vi "ZenReport init.vi"(8 "error IO":errorcluster, 9 "Get part / batch data":variant, 11 "Report type":string(combo)="Part") -> (0 "Error out":errorcluster, 3 "output cluster":T1)   [LabVIEW 2015]
uses:
  Typedefs/ZenReport internal data.ctl
  Typedefs/System configuration.ctl
  Typedefs/Part configuration.ctl
  Typedefs/Batch configuration.ctl
  Typedefs/Internal data.ctl
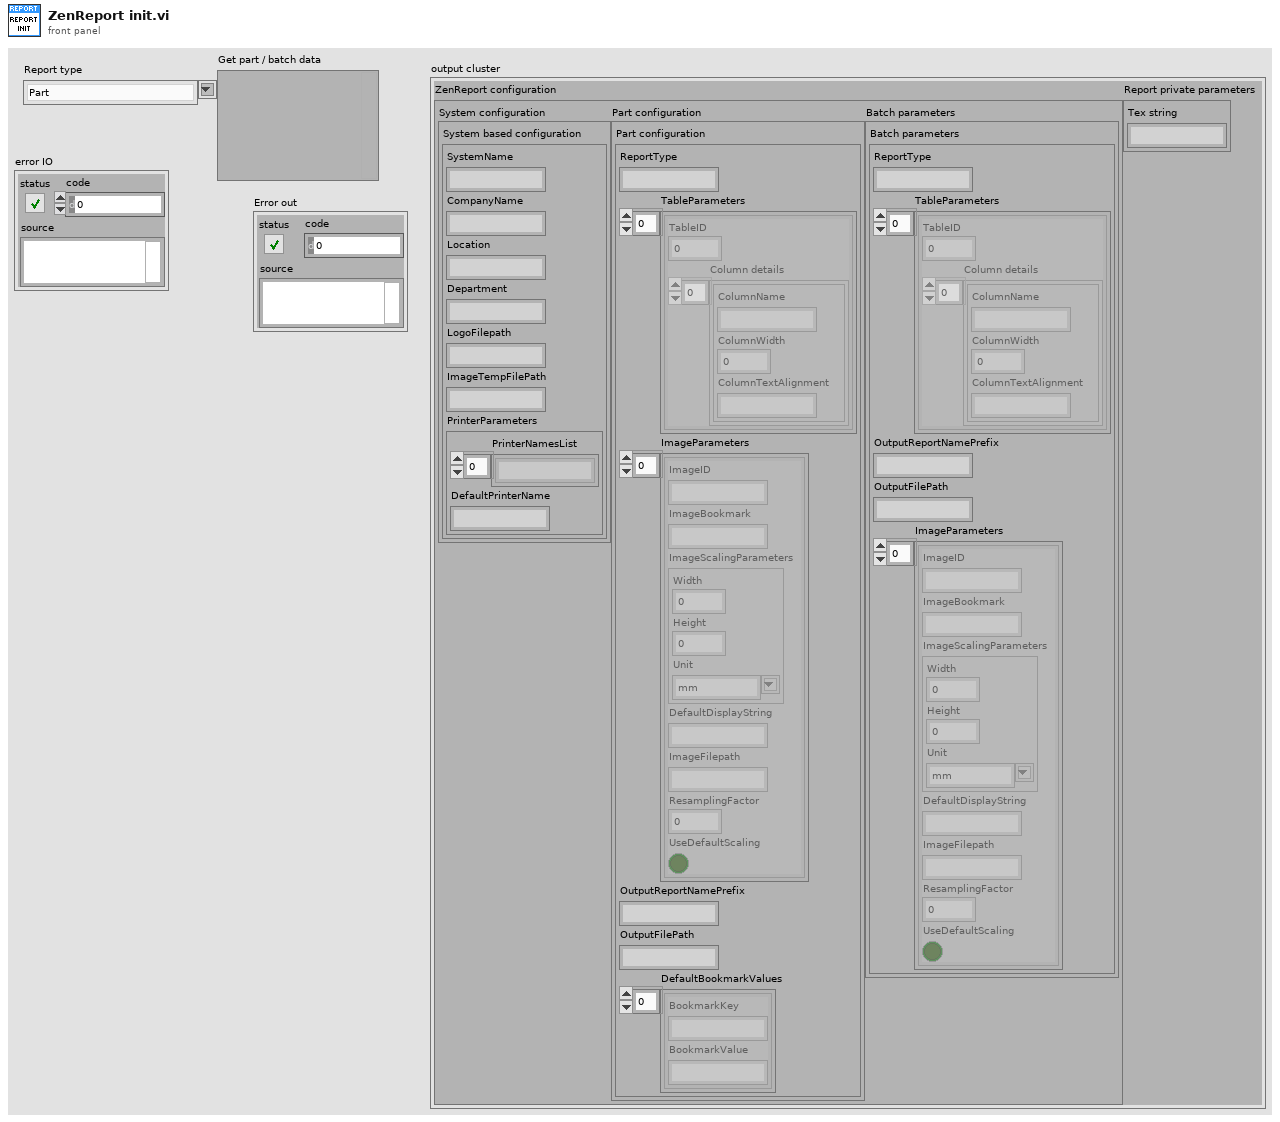
[diagram p1: front panel]
types:
  T1 = typedef "ZenReport internal data.ctl" = cluster{"ZenReport configuration":cluster{"System configuration":T2, "Part configuration":T3, "Batch parameters":T4}, "Report private parameters":T5}
  T2 = typedef "System configuration.ctl" = cluster{"System based configuration":cluster{"SystemName":string, "CompanyName":string, "Location":string, "Department":string, "LogoFilepath":string, "ImageTempFilePath":string, "PrinterParameters":cluster{"PrinterNamesList":string[], "DefaultPrinterName":string}}}
  T3 = typedef "Part configuration.ctl" = cluster{"Part configuration":cluster{"ReportType":string, "TableParameters":cluster{"TableID":dbl, "Column details":cluster{"ColumnName":string, "ColumnWidth":dbl, "ColumnTextAlignment":string}[]}[], "ImageParameters":cluster{"ImageID":string, "ImageBookmark":string, "ImageScalingParameters":cluster{"Width":u32, "Height":u32, "Unit":string}, "DefaultDisplayString":string, "ImageFilepath":string, "ResamplingFactor":dbl, "UseDefaultScaling":bool}[], "OutputReportNamePrefix":string, "OutputFilePath":string, "DefaultBookmarkValues":cluster{"BookmarkKey":string, "BookmarkValue":string}[]}}
  T4 = typedef "Batch configuration.ctl" = cluster{"Batch parameters":cluster{"ReportType":string, "TableParameters":cluster{"TableID":dbl, "Column details":cluster{"ColumnName":string, "ColumnWidth":dbl, "ColumnTextAlignment":string}[]}[], "OutputReportNamePrefix":string, "OutputFilePath":string, "ImageParameters":cluster{"ImageID":string, "ImageBookmark":string, "ImageScalingParameters":cluster{"Width":u32, "Height":u32, "Unit":string}, "DefaultDisplayString":string, "ImageFilepath":string, "ResamplingFactor":dbl, "UseDefaultScaling":bool}[]}}
  T5 = typedef "Internal data.ctl" = cluster{"Tex string":string}
  T6 = cluster{"Error code":i32, "Error details":string}[]
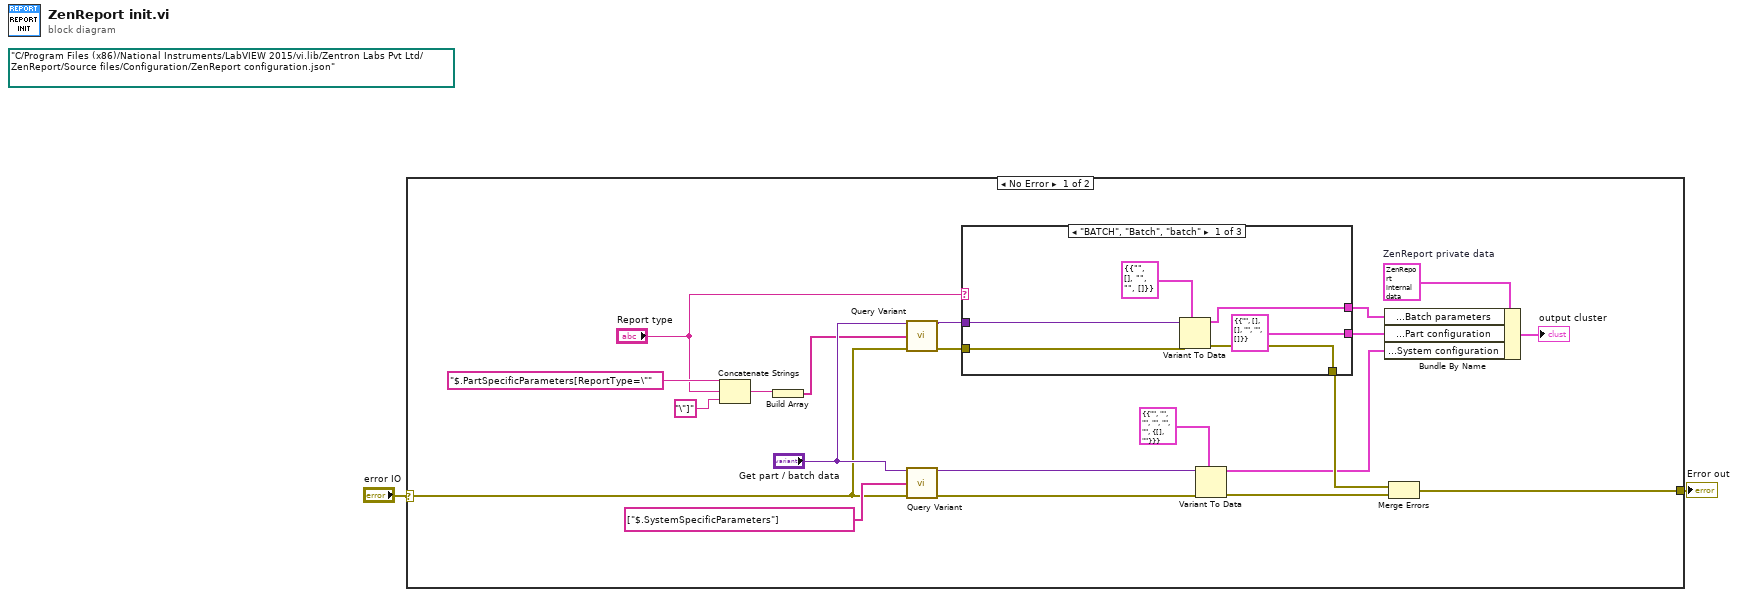
[diagram p0: block diagram]
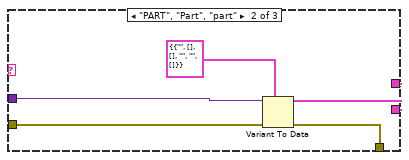
[diagram p2: hidden frame]
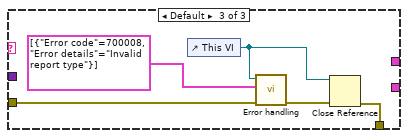
[diagram p3: hidden frame]
diagram:
  (unwired) path "C:/Program Files (x86)/National Instruments/LabVIEW 2015/vi.lib/Zentron Labs Pvt Ltd/ZenReport/Source files/Configuration/ZenReport configuration.json" ("JSON FilePath")
  n1 = case shown="No Error" "error IO" {
    selector: "error IO" -> [w4 w41]
    tunnel: [w3 w41] -> w2
    frame No Error {
      w17 = T1 {"ZenReport configuration"={"System configuration"={"System based configuration"={"SystemName"="", "CompanyName"="", "Location"="", "Department"="", "LogoFilepath"="", "ImageTempFilePath"="", "PrinterParameters"={"PrinterNamesList"=[], "DefaultPrinterName"=""}}}, "Part configuration"={"Part configuration"={"ReportType"="", "TableParameters"=[], "ImageParameters"=[], "OutputReportNamePrefix"="", "OutputFilePath"="", "DefaultBookmarkValues"=[]}}, "Batch parameters"={"Batch parameters"={"ReportType"="", "TableParameters"=[], "OutputReportNamePrefix"="", "OutputFilePath"="", "ImageParameters"=[]}}}, "Report private parameters"={"Tex string"=""}}  # ZenReport private data
      n2 = Concatenate Strings("$.PartSpecificParameters[ReportType=\"", "Report type", "\"]" ("string")) -> (w10:string)
      n3 = Build Array(w10) -> (w9:string[])
      n4 = call <vilib>:"Query Variant.vi"("VCluster in"="Get part / batch data", "pathList"=w9, "error IO"=w4) -> ("VCluster\n out"=w5:variant, "error out"=w6:errorcluster)  [unwired: 9 in, 2 out]
      n5 = call <vilib>:"Query Variant.vi"("VCluster in"="Get part / batch data", "pathList"=string[] ["$.SystemSpecificParameters"], "error IO"=w4) -> ("VCluster\n out"=w8:variant, "error out"=w15:errorcluster)  [unwired: 9 in, 2 out]
      n6 = case shown="\"BATCH\", \"Batch\", \"batch\"" "Report type" {
        tunnel: w6 -> [w29 w35 w39]
        tunnel: [w28 w34 w37] -> w21
        tunnel: w5 -> [w27 w33 _]
        tunnel: [T3 {"Part configuration"={"ReportType"="", "TableParameters"=[], "ImageParameters"=[], "OutputReportNamePrefix"="", "OutputFilePath"="", "DefaultBookmarkValues"=[]}} ("Part parameters") w32 _] -> w20
        tunnel: [w26 w31 _] -> w19
        frame "BATCH", "Batch", "batch" {
          n7 = Variant To Data(error in=w29, type=T4 {"Batch parameters"={"ReportType"="", "TableParameters"=[], "OutputReportNamePrefix"="", "OutputFilePath"="", "ImageParameters"=[]}} ("Batch parameters"), Variant=w27) -> (data=w26:T4, error out=w28:errorcluster)
        }
        frame "PART", "Part", "part" {
          w31 = T4 {"Batch parameters"={"ReportType"="", "TableParameters"=[], "OutputReportNamePrefix"="", "OutputFilePath"="", "ImageParameters"=[]}}  # Batch parameters
          n8 = Variant To Data(error in=w35, type=T3 {"Part configuration"={"ReportType"="", "TableParameters"=[], "ImageParameters"=[], "OutputReportNamePrefix"="", "OutputFilePath"="", "DefaultBookmarkValues"=[]}} ("Part configuration"), Variant=w33) -> (data=w32:T3, error out=w34:errorcluster)
        }
        frame Default {
          n9 = control-ref of="This VI"() -> (w40:refnum<vi>)
          n10 = call "Error handling.vi"("error in"=w39, "User defined error array"=T6 [{"Error code"=700008, "Error details"="Invalid report type"}], "VI reference"=w40) -> ("error IO"=w38:errorcluster)  [unwired: 7 in, 1 out]
          n11 = Close Reference(reference=w40, error in (no error)=w38) -> (error out=w37:errorcluster)
        }
      }
      n12 = Variant To Data(error in=w15, type=T2 {"System based configuration"={"SystemName"="", "CompanyName"="", "Location"="", "Department"="", "LogoFilepath"="", "ImageTempFilePath"="", "PrinterParameters"={"PrinterNamesList"=[], "DefaultPrinterName"=""}}} ("System configuration"), Variant=w8) -> (data=w18:T2, error out=w22:errorcluster)
      n13 = Bundle By Name(cluster=w17, "ZenReport configuration.Batch parameters"=w19, "ZenReport configuration.Part configuration"=w20, "ZenReport configuration.System configuration"=w18) -> (→"output cluster":T1)
      n14 = Merge Errors(w21, w22) -> (w3:errorcluster)
    }
    frame Error {
    }
  }
  "Error out" <- w2
